vi "Latch Timeout with registered input and output.vi"(9 "Timeout?":bool, 10 "Clear":bool) -> (1 "Ever Timed Out?":bool)   [LabVIEW 2011]
uses:
  <vilib>/rvi/FXPMathLib/basic elements/FxpDiscreteDelay/XNode/nifxpmath_DiscreteDelay.xnode
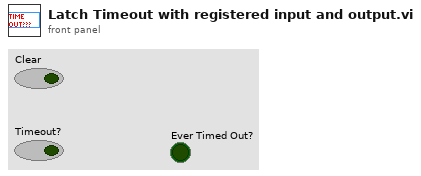
[diagram p1: front panel]
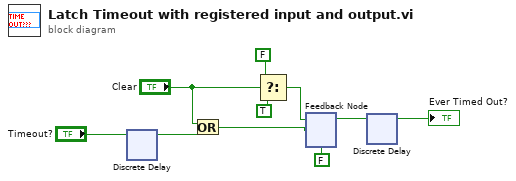
[diagram p0: block diagram]
diagram:
  n1 = xnode "Discrete Delay"("D"="Timeout?") -> ("Q"=w2:bool)
  n2 = Or(x="Clear", y=w2) -> (x .or. y?=w7:bool)
  n3 = Select(t=FALSE, s="Clear", f=TRUE) -> (s? t:f=w3:bool)
  n4 = feedback #1(FALSE) -> (w9:bool)
  n5 = feedback-in #1(w3, w7) -> ()
  n6 = xnode "Discrete Delay"("D"=w9) -> ("Q"=→"Ever Timed Out?":bool)
